vi "testBOOLEAN Failes If Element Is Not Found.vi"(8 "error in (no error)":errorcluster, 11 "TestCase in":refnum<class "Search In 1D Array Test Case.lvclass">) -> (0 "error out":errorcluster, 3 "TestCase out":refnum<class "Search In 1D Array Test Case.lvclass">)   [LabVIEW 2015, in "Search In 1D Array Test Case.lvclass"]
uses:
  Search In 1D Array Test Case.lvclass
  SubVIs/Search in array/Pass If In 1D Array (BOOLEAN).vi
  <vilib>/addons/_JKI Toolkits/VI Tester/TestCase.llb/TestCase.lvclass
  VITAC.lvlib
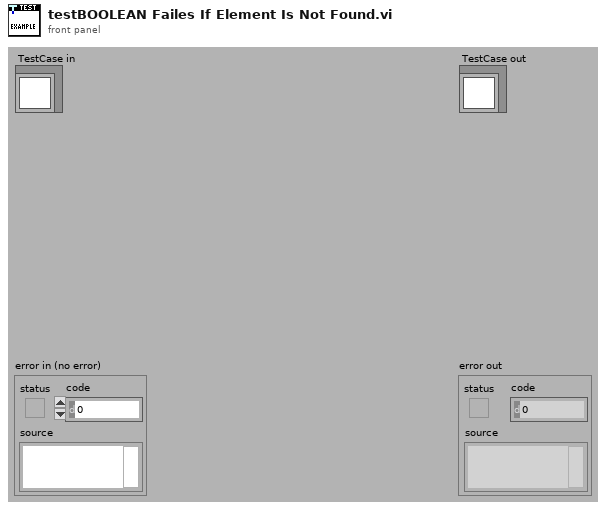
[diagram p1: front panel]
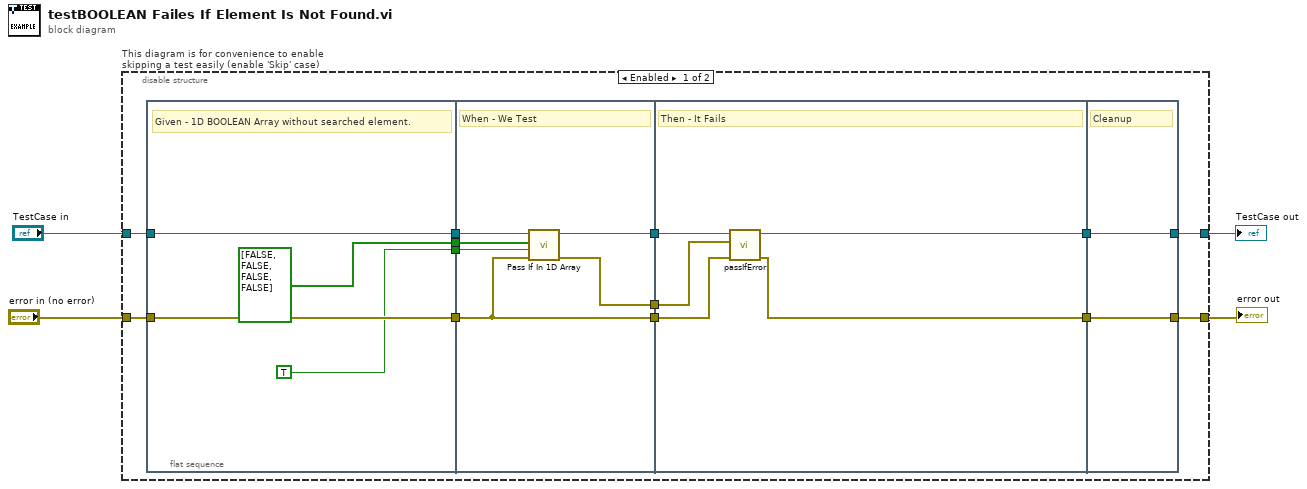
[diagram p0: block diagram]
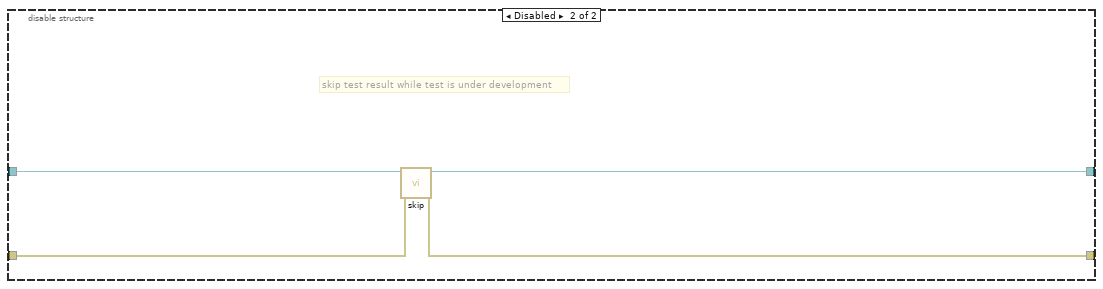
[diagram p2: hidden frame]
diagram:
  n1 = disable-structure "This diagram is for convenience to enable skipping a test easily (enable 'Skip' case)" shown="Enabled" {
    disable-tunnel: "TestCase in" -> [w9 w38]
    disable-tunnel: [w12 w36] -> w1
    disable-tunnel: [w11 w37] -> w3
    disable-tunnel: "error in (no error)" -> [w10 w35]
    frame Enabled {
      n2 = flat-sequence {
        tunnel: w10 -> [w20]
        tunnel: w9 -> [w21]
        tunnel: [w21] -> w17
        tunnel: [w20] -> w16
        tunnel: [TRUE] -> w8
        tunnel: [bool[] [FALSE, FALSE, FALSE, FALSE]] -> w7
        tunnel: [w26] -> w15
        tunnel: [w25] -> w14
        tunnel: w17 -> [w27]
        tunnel: w16 -> [w22]
        tunnel: w8 -> [w24]
        tunnel: w7 -> [w23]
        tunnel: [w22] -> w6
        tunnel: [w32] -> w13
        tunnel: w15 -> [w30]
        tunnel: w14 -> [w29]
        tunnel: w6 -> [w28]
        tunnel: [w31] -> w5
        tunnel: [w33] -> w11
        tunnel: [w34] -> w12
        tunnel: w13 -> [w34]
        tunnel: w5 -> [w33]
        frame #0 {
          # "Given - 1D BOOLEAN Array without searched element."
        }
        frame #1 {
          # "When - We Test"
          n3 = call-poly "Pass If In 1D Array.vi"("error in (no error)"=w22, "element"=w24, "1D array"=w23, "TestCase in"=w27) -> ("error out"=w25:errorcluster, "TestCase out"=w26:refnum<class "Search In 1D Array Test Case.lvclass">)  [unwired: 6 in]
        }
        frame #2 {
          # "Then - It Fails"
          n4 = call-dynamic "passIfError.vi"("error in (no error)"=w28, "error"=w29, "TestCase in"=w30) -> ("error out"=w31:errorcluster, "TestCase out"=w32:refnum<class "Search In 1D Array Test Case.lvclass">)  [unwired: 7 in]
        }
        frame #3 {
          # "Cleanup"
        }
      }
    }
    frame Disabled {
      # "skip test result while test is under development"
      n5 = call <vilib>:"skip.vi"("error in (no error)"=w35, "TestCase in"=w38) -> ("error out"=w37:errorcluster, "TestCase out"=w36:refnum<class "Search In 1D Array Test Case.lvclass">)  [unwired: 8 in]
    }
  }
  "error out" <- w3
  "TestCase out" <- w1
